vi "CDMA_TxCRCattach.vi"(8 "error in (no error)":errorcluster caption="错误输入（无错误）", 9 "crc_num":dbl, 10 "pdch_data":dbl[](array[numeric]), 11 "Path":path) -> (0 "error out":errorcluster caption="错误输出", 2 "attach_crc_data":dbl[](array[numeric]), 3 "Path Out":path)   [LabVIEW 2015]
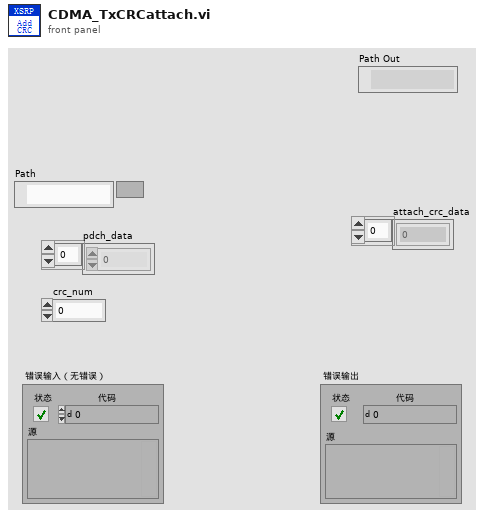
[diagram p1: front panel]
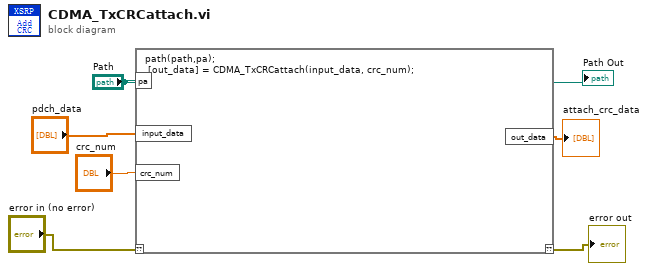
[diagram p0: block diagram]
diagram:
  n1 = script code="path(path,pa);\n [out_data] = CDMA_TxCRCattach(input_data, crc_num);"("??"="error in (no error)", "pa"="Path", "input_data"="pdch_data", "crc_num"="crc_num") -> ("??"=→"error out":errorcluster, "out_data"=→"attach_crc_data":dbl[])
  "Path Out" <- "Path"
